vi "Color Sensor V3 Add Color Match.vi"(10 "Color":cluster{"R":dbl, "G":dbl, "B":dbl}, 11 "Name":string) -> ()   [LabVIEW 2023]
uses:
  Typedef/Color Sensor V3 Color Match.ctl
  Typedef/Color Sensor V3 FGV Command.ctl
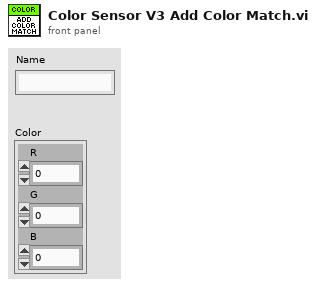
[diagram p1: front panel]
types:
  T1 = typedef "Color Sensor V3 FGV Command.ctl" = enum16{"Update", "Read"}
  T2 = typedef "Color Sensor V3 Color Match.ctl" = cluster{"Name":string, "Color":cluster{"R":dbl, "G":dbl, "B":dbl}}
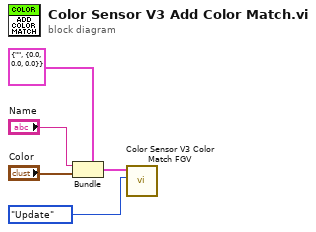
[diagram p0: block diagram]
diagram:
  n1 = Bundle(cluster=T2 {"Name"="", "Color"={"R"=0.0, "G"=0.0, "B"=0.0}} ("output cluster"), "Name"="Name", "Color"="Color") -> (w3:T2)
  n2 = call "Color Sensor V3 Color Match FGV.vi"("FGV Cmd"=Color_Sensor_V3_FGV_Command."Update" ("ColorMatchFGV-Cmd"), "Color Match"=w3) -> ()  [unwired: 9 in, 1 out]
